vi "TCP- Server- 1.vi"() -> ()   [LabVIEW 2015]
doc: "Demonstrates how to use network streams to pass data and commands between two running VIs. It displays waveform data that is received from the target VI and sends commands to update the frequency of the generated signal."
panel:
  in  "Cluster":cluster{"Frequency":i32}={"Frequency"=10}
  in  "Server Closed":string="The server VI closed the connection."
  out "value":T1
  in  "Client Closed":string="The client VI closed the connection."
  in  "Stop":bool
  # "Overview: Demonstrates how to use Network Streams to pass data and commands between two running VIs.\nRequirements: Windows\nInstructions:\n1. Make sure Simple Network Streams - Target.vi is already running.\n2. Run this VI.\n3. Change the Frequency value and observe the change in data that results from sending the new frequency value to the Target VI.\n4. Change the Read Speed value in this VI, and the Write Speed value in the Target VI, and observe the resulting values of Available Elements to Read and Available Elements to Write.\n5. Click Stop to stop the VI."
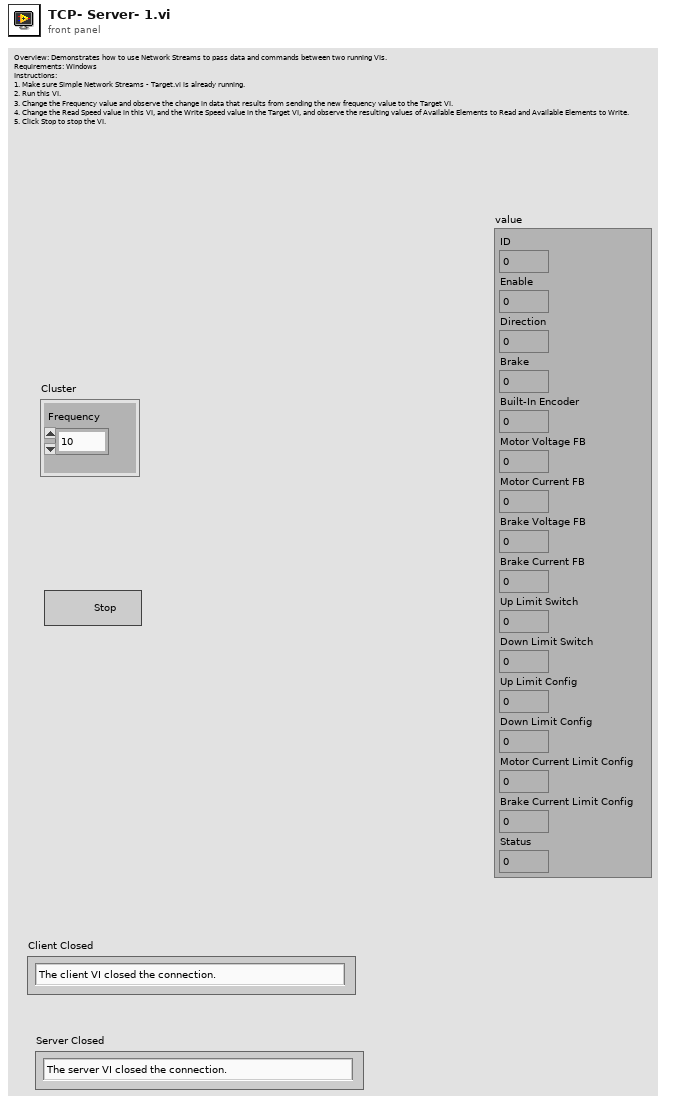
[diagram p1: front panel]
types:
  T1 = cluster{"ID":dbl, "Enable":dbl, "Direction":dbl, "Brake":dbl, "Built-In Encoder":dbl, "Motor Voltage FB":dbl, "Motor Current FB":dbl, "Brake Voltage FB":dbl, "Brake Current FB":dbl, "Up Limit Switch":dbl, "Down Limit Switch":dbl, "Up Limit Config":dbl, "Down Limit Config":dbl, "Motor Current Limit Config":dbl, "Brake Current Limit Config":dbl, "Status":dbl}
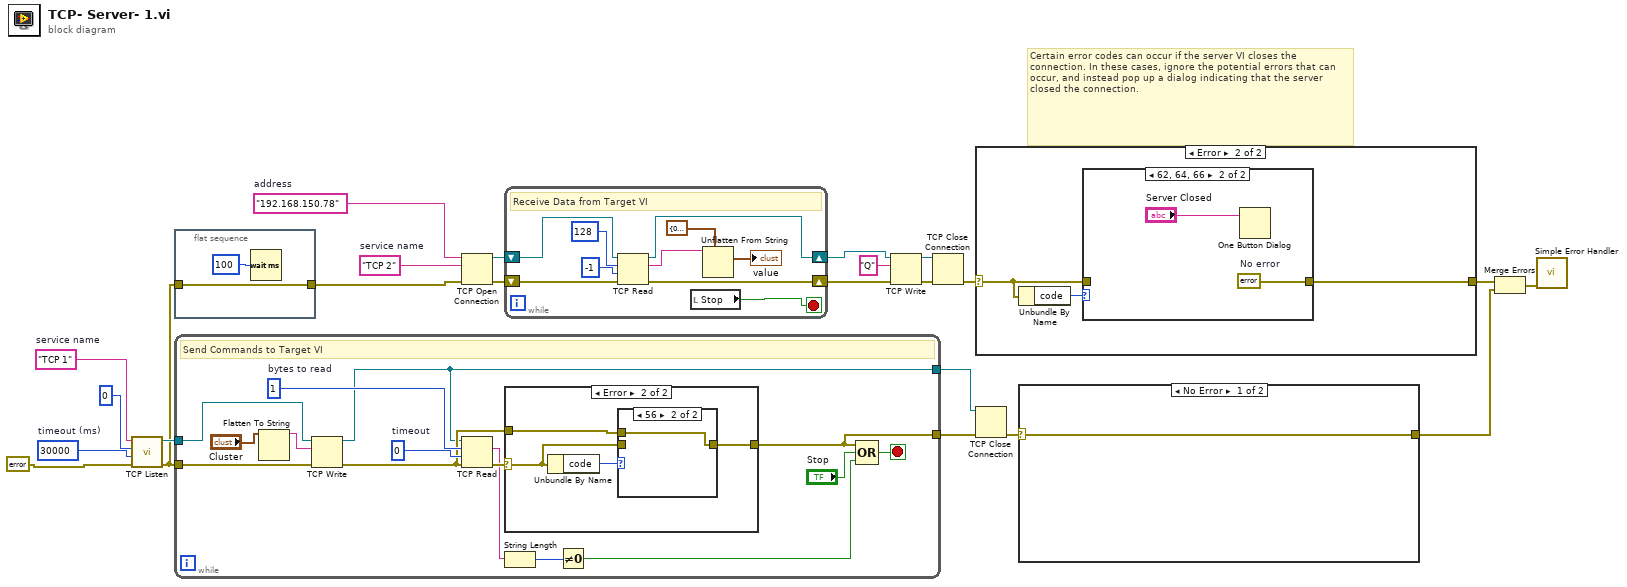
[diagram p0: block diagram]
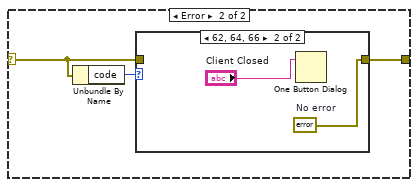
[diagram p4: hidden frame]
diagram:
  w4 = "TCP 2"  # service name
  w16 = "192.168.150.78"  # address
  w22 = "TCP 1"  # service name
  w21 = 30000  # timeout (ms)
  # "Certain error codes can occur if the server VI closes the connection. In these cases, ignore the potential errors that can occur, and instead pop up a dialog indicating that the server closed the connection."
  n1 = call <vilib>:"TCP Listen.vi"("error in (no error)"=errorcluster {"status"=FALSE, "code"=0, "source"=""} ("error out"), "timeout ms (wait forever: -1)"=w21, "port"=u16 0, "service name"=w22) -> ("error out"=w1:errorcluster, "connection ID"=w20:refnum<k5>)  [unwired: 3 in, 3 out]
  n2 = flat-sequence {
    tunnel: w1 -> [w24]
    tunnel: [w24] -> w2
    frame #0 {
      n3 = Wait (ms)(milliseconds to wait=u32 100) -> ()  [unwired: 1 out]
    }
  }
  n4 = while "Host->Target Command Writer" {
    tunnel: w1 -> [w40]
    tunnel: w20 -> [w29]
    tunnel: [w31] -> w18
    tunnel: [w30] -> w17
    stop <- w33 stop-if-true
    w36 = 0  # timeout
    w35 = 1  # bytes to read
    # "Send Commands to Target VI"
    n5 = Flatten To String(anything="Cluster") -> (data string=w27:string)  [unwired: 3 in, 2 out]
    n6 = TCP Write(connection ID=w29, data in=w27, error in (no error)=w40) -> (connection ID out=w30:refnum<k5>, error out=w34:errorcluster)  [unwired: 2 out]
    n7 = TCP Read(connection ID=w30, bytes to read=w35, error in (no error)=w34, 9:w36) -> (data out=w38:string, error out=w39:errorcluster)  [unwired: 2 out]
    n8 = case shown="Error" w39 {
      selector: w39 -> [w41 w44]
      tunnel: [w41 w42] -> w31
      tunnel: w34 -> [_ w43]
      frame No Error {
      }
      frame Error {
        n9 = Unbundle By Name(w44) -> ("code"=w45:i32)
        n10 = case shown="56" w45 {
          tunnel: w44 -> [w46 _]
          tunnel: w43 -> [_ w47]
          tunnel: [w46 w47] -> w42
          frame Default {
          }
          frame 56 {
          }
        }
      }
    }
    n11 = String Length(string=w38) -> (length=w37:i32)
    n12 = Not Equal To 0?(x=w37) -> (x != 0?=w32:bool)
    n13 = Compound Arithmetic op=OR(w31, "Stop", w32) -> (w33:bool)
  }
  n14 = TCP Open Connection(address=w16, remote port or service name=w4, error in (no error)=w2) -> (connection ID=w14:refnum<k5>, error out=w15:errorcluster)  [unwired: 2 in]
  n15 = while "Target->Host Data Reader" {
    shift-right: [w51] -> w8
    shift-left: w15 -> [w52]
    shift-right: [w50] -> w7
    shift-left: w14 -> [w49]
    stop <- w48 stop-if-true
    # "Receive Data from Target VI"
    n16 = TCP Read(connection ID=w49, bytes to read=128, error in (no error)=w52, 9:-1 ("timeout ms (25000)")) -> (connection ID out=w50:refnum<k5>, data out=w55:string, error out=w51:errorcluster)  [unwired: 1 in]
    n17 = local read "Stop"() -> (w48:bool)
    n18 = Unflatten From String(type=T1 {"ID"=0.0, "Enable"=0.0, "Direction"=0.0, "Brake"=0.0, "Built-In Encoder"=0.0, "Motor Voltage FB"=0.0, "Motor Current FB"=0.0, "Brake Voltage FB"=0.0, "Brake Current FB"=0.0, "Up Limit Switch"=0.0, "Down Limit Switch"=0.0, "Up Limit Config"=0.0, "Down Limit Config"=0.0, "Motor Current Limit Config"=0.0, "Brake Current Limit Config"=0.0, "Status"=0.0} ("MirrorCoverMotor"), binary string=w55) -> (value=→"value":T1)  [unwired: 3 in, 2 out]
  }
  n19 = TCP Write(connection ID=w7, data in="Q", error in (no error)=w8) -> (connection ID out=w9:refnum<k5>, error out=w10:errorcluster)  [unwired: 2 out]
  n20 = TCP Close Connection(connection ID=w9, error in (no error)=w10) -> (error out=w12:errorcluster)  [unwired: 1 in, 1 out]
  n21 = case shown="Error" w12 {
    selector: w12 -> [w58 w60]
    tunnel: [w58 w59] -> w6
    frame No Error {
    }
    frame Error {
      n22 = Unbundle By Name(w60) -> ("code"=w61:i32)
      n23 = case shown="62, 64, 66" w61 {
        tunnel: w60 -> [w62 _]
        tunnel: [w62 w64] -> w59
        frame Default {
        }
        frame 62, 64, 66 {
          w64 = errorcluster {"status"=FALSE, "code"=0, "source"=""}  # No error
          n24 = One Button Dialog(message="Server Closed") -> ()  [unwired: 1 in, 1 out]
        }
      }
    }
  }
  n25 = TCP Close Connection(connection ID=w17, error in (no error)=w18) -> (error out=w19:errorcluster)  [unwired: 2 out]
  n26 = case shown="No Error" w19 {
    selector: w19 -> [w65 w67]
    tunnel: [w65 w66] -> w5
    frame No Error {
    }
    frame Error {
      n27 = Unbundle By Name(w67) -> ("code"=w68:i32)
      n28 = case shown="62, 64, 66" w68 {
        tunnel: w67 -> [w69 _]
        tunnel: [w69 w71] -> w66
        frame Default {
        }
        frame 62, 64, 66 {
          w71 = errorcluster {"status"=FALSE, "code"=0, "source"=""}  # No error
          n29 = One Button Dialog(message="Client Closed") -> ()  [unwired: 1 in, 1 out]
        }
      }
    }
  }
  n30 = Merge Errors(w6, w5) -> (w23:errorcluster)
  n31 = call <vilib>:"Simple Error Handler.vi"("error in (no error)"=w23) -> ()  [unwired: 4 in, 5 out]
